vi "Unflatten UIP Value.vi"(10 "String Value":string, 11 "FontUIP In":refnum<class "FontUIP.lvclass">) -> (0 "Error Out":errorcluster, 3 "FontUIP Out":refnum<class "FontUIP.lvclass">)   [LabVIEW 2016, in "FontUIP.lvclass"]
doc: "Overwrite this abstract method to implement child behavior for unflattening the UIP private data from XML compatible string format."
uses:
  FontUIP.lvclass
  <vilib>/Utility/miscctls.llb/LVFontTypeDef.ctl
  FontUIP.lvclass/FontUIP.ctl
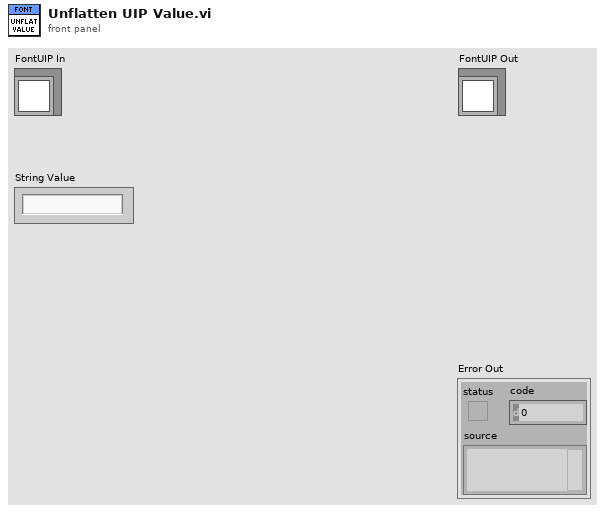
[diagram p1: front panel]
types:
  T1 = typedef "LVFontTypeDef.ctl" = cluster{"Font Name":string, "Size":u16, "Bold":bool, "Italic":bool, "Underline":bool, "Strikeout":bool, "Color":u32}
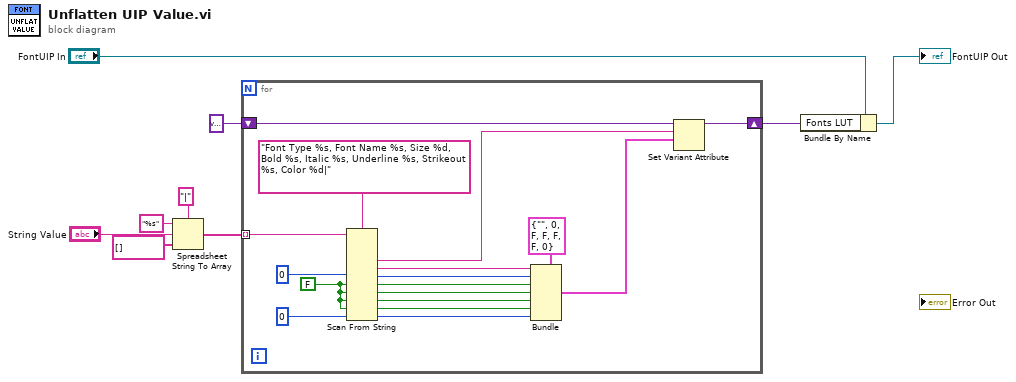
[diagram p0: block diagram]
diagram:
  n1 = Spreadsheet String To Array(delimiter (Tab)="|", format string="%s", spreadsheet string="String Value", array type (2D Dbl)=string[] []) -> (array=w4:string[])
  n2 = for {
    tunnel: w4 -> [w26] mode=indexing
    shift-right: [w24] -> w1
    shift-left: variant -> [w23]
    w12 = FALSE
    n3 = Scan From String(format string="Font Type %s, Font Name %s, Size %d, Bold %s, Italic %s, Underline %s, Strikeout %s, Color %d|", input string=w26, default 3=u16 0, default 4=w12, default 5=w12, default 6=w12, default 7=w12, default 8=u32 0) -> (output 1=w22:string, output 2=w20:string, output 3=w19:u16, output 4=w18:bool, output 5=w17:bool, output 6=w16:bool, output 7=w15:bool, output 8=w14:u32)  [unwired: 4 in, 3 out]
    n4 = Bundle(cluster=T1 {"Font Name"="", "Size"=0, "Bold"=FALSE, "Italic"=FALSE, "Underline"=FALSE, "Strikeout"=FALSE, "Color"=0} ("Font out"), "Font Name"=w20, "Size"=w19, "Bold"=w18, "Italic"=w17, "Underline"=w16, "Strikeout"=w15, "Color"=w14) -> (w10:T1)
    n5 = Set Variant Attribute(Variant=w23, name=w22, value=w10) -> (Variant out=w24:variant)  [unwired: 1 in, 2 out]
  }
  n6 = Bundle By Name(cluster="FontUIP In", "Fonts LUT"=w1) -> (→"FontUIP Out":refnum<class "FontUIP.lvclass">)
